vi "globalSetUp.vi"(8 "error in":errorcluster, 11 "Loopback in":refnum<class "Loopback.lvclass">) -> (0 "error out":errorcluster, 3 "Loopback out":refnum<class "Loopback.lvclass">)   [LabVIEW 2020, in "Loopback.lvclass"]
uses:
  Loopback.lvclass
  Shared/Device Parameters.ctl
  Shared/Initialization Method.ctl
  Loopback.lvclass/Loopback.ctl
  niveristand-custom-device-testing-tools/VeriStandTestUtilities/VeriStandTestUtilities.lvlib
  Scripting/Ballard MIL-STD-1553 Scripting.lvlib
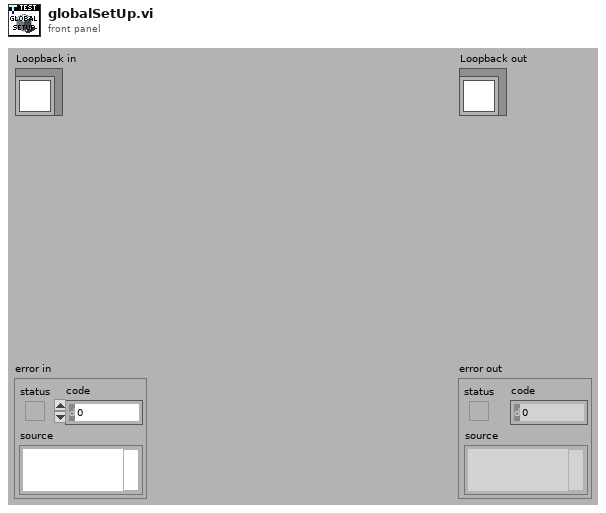
[diagram p1: front panel]
types:
  T1 = typedef "Device Parameters.ctl" = cluster{"initialization method":T2, "card number":i32, "PXI slot number":i32, "core number":i32}
  T2 = typedef "Initialization Method.ctl" = enum16{"PXI Slot Number", "Card Number"}
  T3 = typedef "Custom Device API.lvlib/Custom Device Item Ref.ctl" = u64
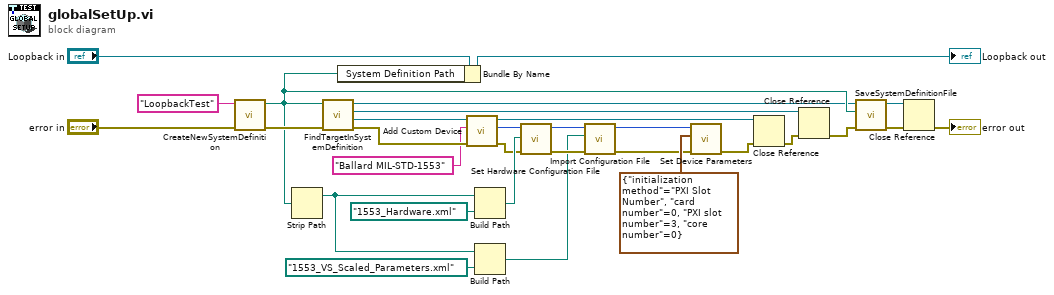
[diagram p0: block diagram]
diagram:
  n1 = call "CreateNewSystemDefinition.vi"("error in"="error in", "System Definition Name"="LoopbackTest") -> ("error out"=w30:errorcluster, "System Definition Path"=w29:path)  [unwired: 8 in]
  n2 = Strip Path(path=w29) -> (stripped path=w6:path)  [unwired: 1 out]
  n3 = call "FindTargetInSystemDefinition.vi"("error in"=w30, "system definition path"=w29) -> ("error out"=w21:errorcluster, "Target"=w15:refnum<k24>, "Root"=w16:refnum<k24>, "System Definition"=w14:refnum<k24>)  [unwired: 6 in]
  n4 = Bundle By Name(cluster="Loopback in", "System Definition Path"=w29) -> (→"Loopback out":refnum<class "Loopback.lvclass">)
  n5 = call "Add Custom Device.vi"("error in"=w21, "name"="Ballard MIL-STD-1553", "target in"=w15) -> ("error out"=w23:errorcluster, "Ballard MIL-STD 1553 custom device"=w22:T3, "target out"=w18:refnum<k24>)  [unwired: 6 in]
  n6 = Build Path(base path=w6, name or relative path=path "1553_Hardware.xml") -> (appended path=w25:path)
  n7 = Build Path(base path=w6, name or relative path=path "1553_VS_Scaled_Parameters.xml") -> (appended path=w5:path)
  n8 = call "Set Hardware Configuration File.vi"("error in"=w23, "hardware configuration file path"=w25, "Ballard MIL-STD 1553 custom device in"=w22) -> ("error out"=w9:errorcluster, "Ballard MIL-STD 1553 custom device out"=w8:T3)  [unwired: 7 in]
  n9 = call "Import Configuration File.vi"("error in"=w9, "parameters configuration file path"=w5, "Ballard MIL-STD 1553 custom device in"=w8) -> ("error out"=w3:errorcluster, "Ballard MIL-STD 1553 custom device out"=w1:T3)  [unwired: 7 in]
  n10 = call "Set Device Parameters.vi"("error in"=w3, "device parameters"=T1 {"initialization method"=enum."PXI Slot Number", "card number"=0, "PXI slot number"=3, "core number"=0}, "Ballard MIL-STD 1553 custom device in"=w1) -> ("error out"=w2:errorcluster)  [unwired: 7 in, 1 out]
  n11 = Close Reference(reference=w18, error in (no error)=w2) -> (error out=w19:errorcluster)
  n12 = Close Reference(reference=w16, error in (no error)=w19) -> (error out=w17:errorcluster)
  n13 = call "SaveSystemDefinitionFile.vi"("error in (no error)"=w17, "System Definition File in"=w29, "System Definition Reference in"=w14) -> ("error out"=w26:errorcluster, "System Definition Reference out"=w27:refnum<k24>)  [unwired: 7 in]
  n14 = Close Reference(reference=w27, error in (no error)=w26) -> (error out=→"error out":errorcluster)
